vi "Send SysCfg Session.vi"(8 "error in":errorcluster, 11 "Controller in":refnum<class "Controller.lvclass">) -> (0 "error out":errorcluster, 2 "SysCfg Session":refnum<k21>, 3 "Controller out":refnum<class "Controller.lvclass">)   [LabVIEW 2015, in "SMI.lvlib" / "Controller.lvclass"]
uses:
  Controller.lvclass
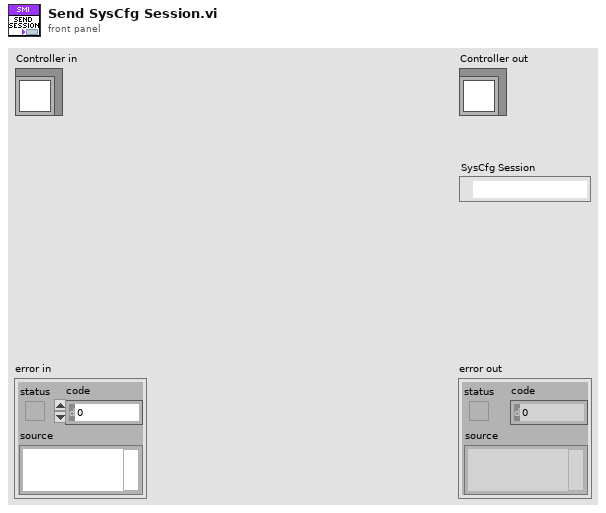
[diagram p1: front panel]
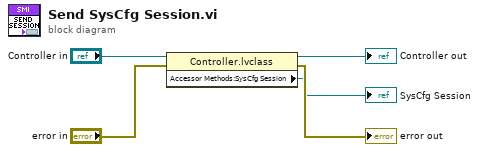
[diagram p0: block diagram]
diagram:
  n1 = property class="Controller.lvclass"(reference="Controller in", error in="error in") -> (reference out=→"Controller out":refnum<class "Controller.lvclass">, error out=→"error out":errorcluster, "Accessor Methods:SysCfg Session"=→"SysCfg Session":refnum<data-value>)
